vi "MDAQ_CalibrationConst.vi"(9 "mV":dbl, 11 "MDU Velocity":dbl) -> (2 "MDAQ V":dbl)   [LabVIEW 2021]
uses:
  <vilib>/Analysis/NI_AALPro.lvlib
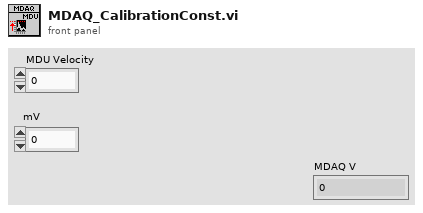
[diagram p1: front panel]
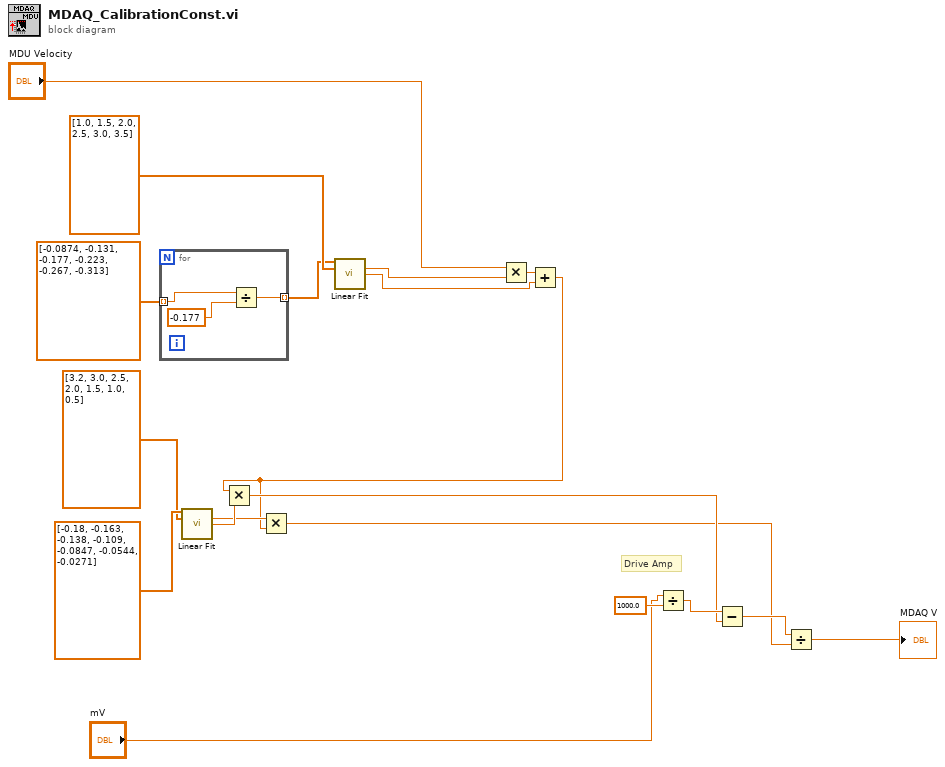
[diagram p0: block diagram]
diagram:
  # "Drive Amp"
  n1 = for {
    tunnel: dbl[] [-0.0874, -0.131, -0.177, -0.223, -0.267, -0.313] -> [w22] mode=indexing
    tunnel: [w20] -> w17 mode=indexing
    n2 = Divide(x=w22, y=-0.177) -> (x/y=w20:dbl)
  }
  n3 = call <vilib>:"Linear Fit.vi"("Y"=dbl[] [-0.18, -0.163, -0.138, -0.109, -0.0847, -0.0544, -0.0271], "X"=dbl[] [3.2, 3.0, 2.5, 2.0, 1.5, 1.0, 0.5]) -> ("slope"=w5:dbl, "intercept"=w8:dbl)  [unwired: 9 in, 3 out]
  n4 = call <vilib>:"Linear Fit.vi"("Y"=w17, "X"=dbl[] [1.0, 1.5, 2.0, 2.5, 3.0, 3.5]) -> ("slope"=w16:dbl, "intercept"=w13:dbl)  [unwired: 9 in, 3 out]
  n5 = Multiply(x="MDU Velocity", y=w16) -> (x*y=w14:dbl)
  n6 = Add(x=w14, y=w13) -> (x+y=w4:dbl)
  n7 = Multiply(x=w4, y=w8) -> (x*y=w7:dbl)
  n8 = Multiply(x=w5, y=w4) -> (x*y=w3:dbl)
  n9 = Divide(x="mV", y=1000.0) -> (x/y=w9:dbl)
  n10 = Subtract(x=w9, y=w7) -> (x-y=w6:dbl)
  n11 = Divide(x=w6, y=w3) -> (x/y=→"MDAQ V":dbl)
